vi "UR5 Dash Commands Test VI.vi"() -> ()   [LabVIEW 2018]
panel:
  in  "Command":string="Load target1.urp"
  in  "Send Command":bool
  in  "Get Loaded Program":bool
  in  "Program Name":string="Load target1.urp"
  in  "Stop Program":bool
  in  "Pause":bool
  in  "Play":bool
  in  "Load Program":bool
  in  "Stop":bool
  out "after substring":string
  out "data out":string
  out "Error Out":errorcluster
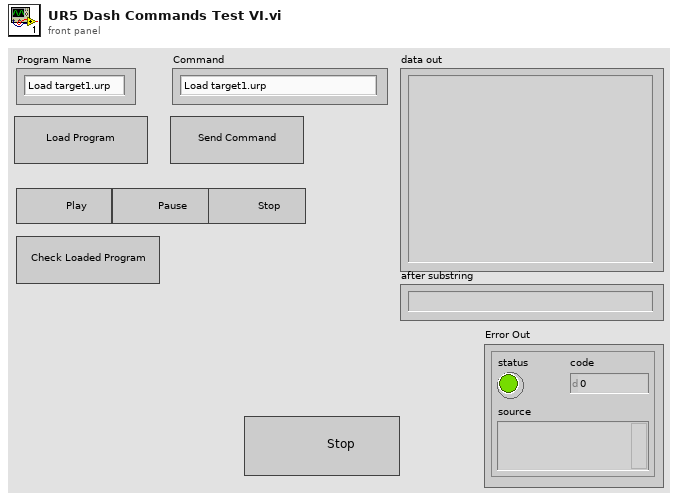
[diagram p1: front panel]
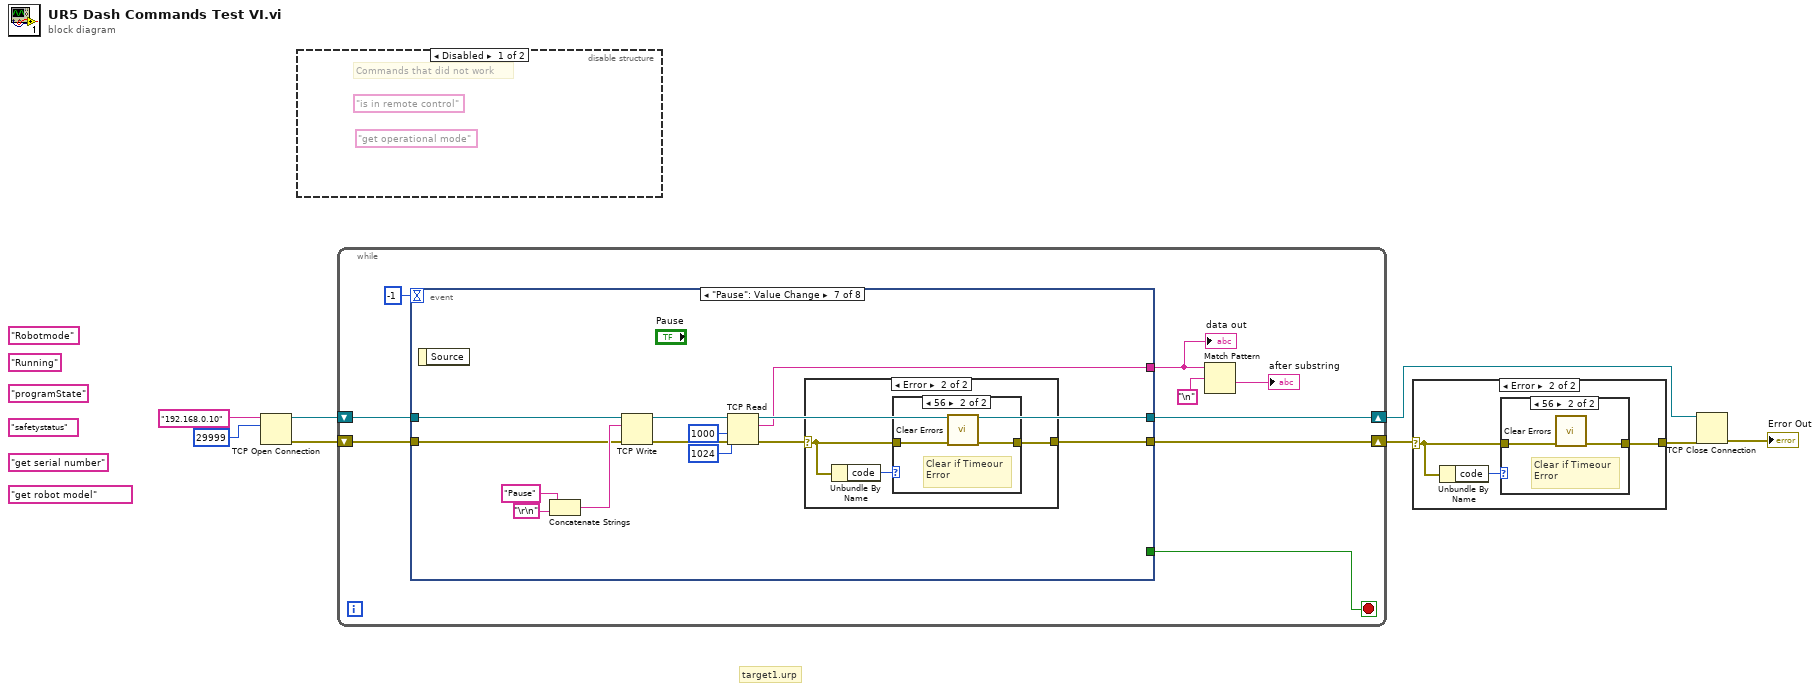
[diagram p0: block diagram]
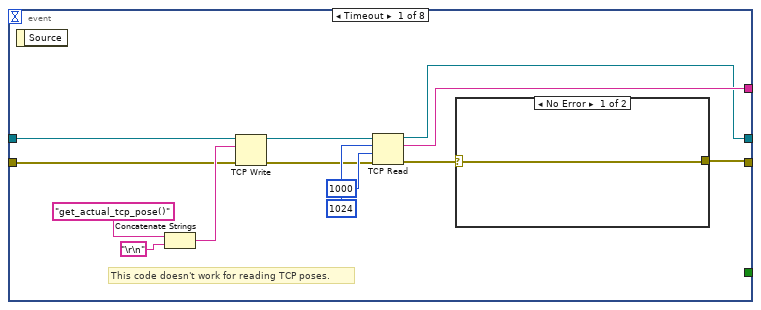
[diagram p4: hidden frame]
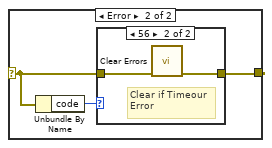
[diagram p5: hidden frame]
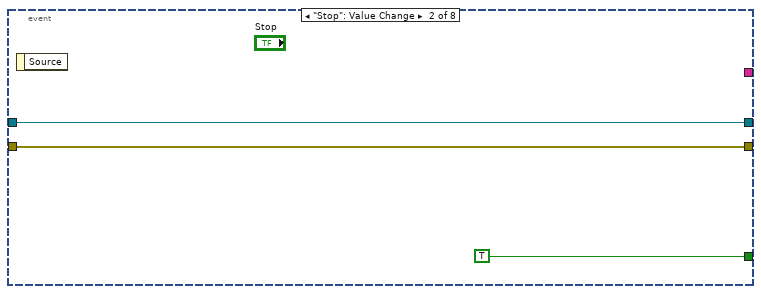
[diagram p7: hidden frame]
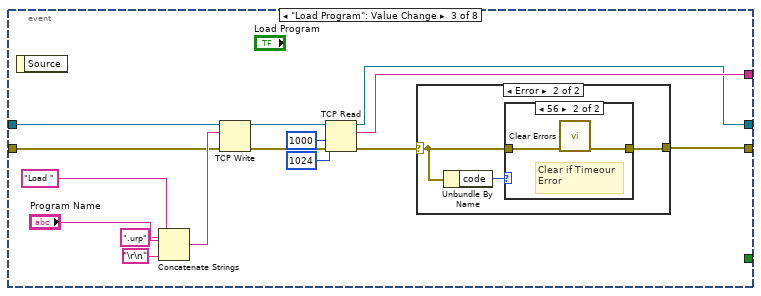
[diagram p8: hidden frame]
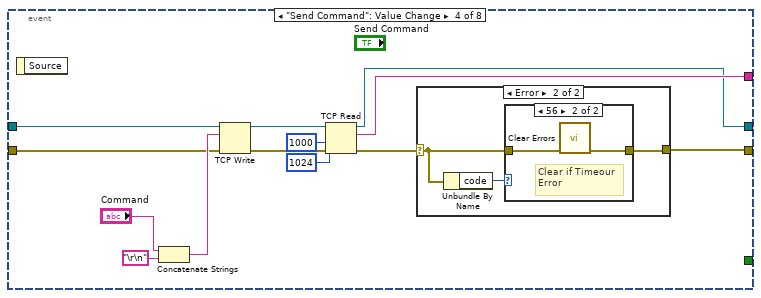
[diagram p11: hidden frame]
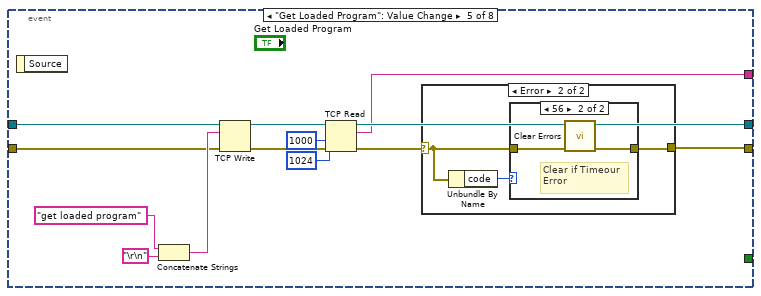
[diagram p14: hidden frame]
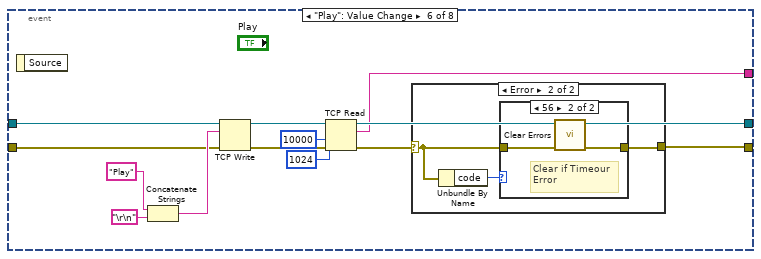
[diagram p17: hidden frame]
diagram:
  (unwired) "Robotmode"
  (unwired) "Running"
  (unwired) "programState"
  (unwired) "safetystatus"
  (unwired) "get serial number"
  (unwired) "get robot model"
  # "target1.urp"
  n1 = TCP Open Connection(address="192.168.0.10", remote port or service name=u16 29999) -> (connection ID=w5:refnum<k5>, error out=w4:errorcluster)  [unwired: 3 in]
  n2 = disable-structure shown="Disabled" {
    frame Disabled {
      (unwired) "get operational mode"
      (unwired) "is in remote control"
      # "Commands that did not work"
    }
    frame Enabled {
    }
  }
  n3 = while {
    shift-right: [w15] -> w1
    shift-left: w5 -> [w16]
    shift-right: [w13] -> w3
    shift-left: w4 -> [w14]
    stop <- w17 stop-if-true
    n4 = event shown="[6] \"Pause\": Value Change" {
      selector: _ -> [_ _ _ _ _ _ _ _]
      dyn-events: _ -> [_ _ _ _ _ _ _ _]
      timeout: -1 -> [_ _ _ _ _ _ _ _]
      tunnel: [_ TRUE _ _ _ _ _ _] -> w17
      tunnel: w16 -> [w23 w39 w49 w69 w89 w109 w129 w149]
      tunnel: [w18 w39 w41 w64 w88 w108 w128 w148] -> w15
      tunnel: [w20 w38 w42 w65 w83 w104 w123 w144] -> w13
      tunnel: w14 -> [w22 w38 w48 w68 w87 w107 w127 w147]
      tunnel: [w19 _ w47 w67 w86 w106 w125 w146] -> w10
      event Timeout {
        # "This code doesn't work for reading TCP poses."
        n5 = event-data() -> ()  [unwired: 1 in, 1 out]
        n6 = Concatenate Strings("get_actual_tcp_pose()" ("string"), "\r\n") -> (w28:string)
        n7 = TCP Write(connection ID=w23, data in=w28, error in (no error)=w22) -> (connection ID out=w30:refnum<k5>, error out=w21:errorcluster)  [unwired: 1 in, 1 out]
        n8 = TCP Read(connection ID=w30, bytes to read=1024, error in (no error)=w21, 9:1000 ("timeout ms (25000)")) -> (connection ID out=w18:refnum<k5>, data out=w19:string, error out=w29:errorcluster)  [unwired: 1 in]
        n9 = case shown="No Error" w29 {
          selector: w29 -> [w31 w33]
          tunnel: [w31 w32] -> w20
          frame No Error {
          }
          frame Error {
            n10 = Unbundle By Name(w33) -> ("code"=w34:i32)
            n11 = case shown="56" w34 {
              tunnel: w33 -> [w35 w37]
              tunnel: [w35 w36] -> w32
              frame 0, Default {
              }
              frame 56 {
                # "Clear if Timeour\nError"
                n12 = call <vilib>:"Clear Errors.vi"("error in (no error)"=w37) -> ("error out"=w36:errorcluster)  [unwired: 5 in, 1 out]
              }
            }
          }
        }
      }
      event "Stop": Value Change {
        n13 = event-data() -> ()  [unwired: 1 in, 1 out]
      }
      event "Load Program": Value Change {
        n14 = event-data() -> ()  [unwired: 1 in, 1 out]
        n15 = Concatenate Strings("Load ", "Program Name", ".urp" ("string"), "\r\n") -> (w53:string)
        n16 = TCP Write(connection ID=w49, data in=w53, error in (no error)=w48) -> (connection ID out=w51:refnum<k5>, error out=w52:errorcluster)  [unwired: 1 in, 1 out]
        n17 = TCP Read(connection ID=w51, bytes to read=1024, error in (no error)=w52, 9:1000 ("timeout ms (25000)")) -> (connection ID out=w41:refnum<k5>, data out=w47:string, error out=w43:errorcluster)  [unwired: 1 in]
        n18 = case shown="Error" w43 {
          selector: w43 -> [w56 w58]
          tunnel: [w56 w57] -> w42
          frame No Error {
          }
          frame Error {
            n19 = Unbundle By Name(w58) -> ("code"=w59:i32)
            n20 = case shown="56" w59 {
              tunnel: w58 -> [w60 w62]
              tunnel: [w60 w61] -> w57
              frame 0, Default {
              }
              frame 56 {
                # "Clear if Timeour\nError"
                n21 = call <vilib>:"Clear Errors.vi"("error in (no error)"=w62) -> ("error out"=w61:errorcluster)  [unwired: 5 in, 1 out]
              }
            }
          }
        }
      }
      event "Send Command": Value Change {
        n22 = event-data() -> ()  [unwired: 1 in, 1 out]
        n23 = Concatenate Strings("Command", "\r\n") -> (w73:string)
        n24 = TCP Write(connection ID=w69, data in=w73, error in (no error)=w68) -> (connection ID out=w71:refnum<k5>, error out=w72:errorcluster)  [unwired: 1 in, 1 out]
        n25 = TCP Read(connection ID=w71, bytes to read=1024, error in (no error)=w72, 9:1000 ("timeout ms (25000)")) -> (connection ID out=w64:refnum<k5>, data out=w67:string, error out=w66:errorcluster)  [unwired: 1 in]
        n26 = case shown="Error" w66 {
          selector: w66 -> [w76 w78]
          tunnel: [w76 w77] -> w65
          frame No Error {
          }
          frame Error {
            n27 = Unbundle By Name(w78) -> ("code"=w79:i32)
            n28 = case shown="56" w79 {
              tunnel: w78 -> [w80 w82]
              tunnel: [w80 w81] -> w77
              frame 0, Default {
              }
              frame 56 {
                # "Clear if Timeour\nError"
                n29 = call <vilib>:"Clear Errors.vi"("error in (no error)"=w82) -> ("error out"=w81:errorcluster)  [unwired: 5 in, 1 out]
              }
            }
          }
        }
      }
      event "Get Loaded Program": Value Change {
        n30 = event-data() -> ()  [unwired: 1 in, 1 out]
        n31 = Concatenate Strings("get loaded program", "\r\n") -> (w93:string)
        n32 = TCP Write(connection ID=w89, data in=w93, error in (no error)=w87) -> (connection ID out=w91:refnum<k5>, error out=w92:errorcluster)  [unwired: 1 in, 1 out]
        n33 = TCP Read(connection ID=w91, bytes to read=1024, error in (no error)=w92, 9:1000 ("timeout ms (25000)")) -> (connection ID out=w88:refnum<k5>, data out=w86:string, error out=w84:errorcluster)  [unwired: 1 in]
        n34 = case shown="Error" w84 {
          selector: w84 -> [w96 w98]
          tunnel: [w96 w97] -> w83
          frame No Error {
          }
          frame Error {
            n35 = Unbundle By Name(w98) -> ("code"=w99:i32)
            n36 = case shown="56" w99 {
              tunnel: w98 -> [w100 w102]
              tunnel: [w100 w101] -> w97
              frame 0, Default {
              }
              frame 56 {
                # "Clear if Timeour\nError"
                n37 = call <vilib>:"Clear Errors.vi"("error in (no error)"=w102) -> ("error out"=w101:errorcluster)  [unwired: 5 in, 1 out]
              }
            }
          }
        }
      }
      event "Play": Value Change {
        n38 = event-data() -> ()  [unwired: 1 in, 1 out]
        n39 = Concatenate Strings("Play", "\r\n") -> (w113:string)
        n40 = TCP Write(connection ID=w109, data in=w113, error in (no error)=w107) -> (connection ID out=w111:refnum<k5>, error out=w112:errorcluster)  [unwired: 1 in, 1 out]
        n41 = TCP Read(connection ID=w111, bytes to read=1024, error in (no error)=w112, 9:10000 ("timeout ms (25000)")) -> (connection ID out=w108:refnum<k5>, data out=w106:string, error out=w105:errorcluster)  [unwired: 1 in]
        n42 = case shown="Error" w105 {
          selector: w105 -> [w116 w118]
          tunnel: [w116 w117] -> w104
          frame No Error {
          }
          frame Error {
            n43 = Unbundle By Name(w118) -> ("code"=w119:i32)
            n44 = case shown="56" w119 {
              tunnel: w118 -> [w120 w122]
              tunnel: [w120 w121] -> w117
              frame 0, Default {
              }
              frame 56 {
                # "Clear if Timeour\nError"
                n45 = call <vilib>:"Clear Errors.vi"("error in (no error)"=w122) -> ("error out"=w121:errorcluster)  [unwired: 5 in, 1 out]
              }
            }
          }
        }
      }
      event "Pause": Value Change {
        n46 = event-data() -> ()  [unwired: 1 in, 1 out]
        n47 = Concatenate Strings("Pause" ("string"), "\r\n") -> (w133:string)
        n48 = TCP Write(connection ID=w129, data in=w133, error in (no error)=w127) -> (connection ID out=w131:refnum<k5>, error out=w132:errorcluster)  [unwired: 1 in, 1 out]
        n49 = TCP Read(connection ID=w131, bytes to read=1024, error in (no error)=w132, 9:1000 ("timeout ms (25000)")) -> (connection ID out=w128:refnum<k5>, data out=w125:string, error out=w124:errorcluster)  [unwired: 1 in]
        n50 = case shown="Error" w124 {
          selector: w124 -> [w136 w138]
          tunnel: [w136 w137] -> w123
          frame No Error {
          }
          frame Error {
            n51 = Unbundle By Name(w138) -> ("code"=w139:i32)
            n52 = case shown="56" w139 {
              tunnel: w138 -> [w140 w142]
              tunnel: [w140 w141] -> w137
              frame 0, Default {
              }
              frame 56 {
                # "Clear if Timeour\nError"
                n53 = call <vilib>:"Clear Errors.vi"("error in (no error)"=w142) -> ("error out"=w141:errorcluster)  [unwired: 5 in, 1 out]
              }
            }
          }
        }
      }
      event "Stop Program": Value Change {
        n54 = event-data() -> ()  [unwired: 1 in, 1 out]
        n55 = Concatenate Strings("Stop", "\r\n") -> (w153:string)
        n56 = TCP Write(connection ID=w149, data in=w153, error in (no error)=w147) -> (connection ID out=w151:refnum<k5>, error out=w152:errorcluster)  [unwired: 1 in, 1 out]
        n57 = TCP Read(connection ID=w151, bytes to read=1024, error in (no error)=w152, 9:1000 ("timeout ms (25000)")) -> (connection ID out=w148:refnum<k5>, data out=w146:string, error out=w143:errorcluster)  [unwired: 1 in]
        n58 = case shown="Error" w143 {
          selector: w143 -> [w156 w158]
          tunnel: [w156 w157] -> w144
          frame No Error {
          }
          frame Error {
            n59 = Unbundle By Name(w158) -> ("code"=w159:i32)
            n60 = case shown="56" w159 {
              tunnel: w158 -> [w160 w162]
              tunnel: [w160 w161] -> w157
              frame 0, Default {
              }
              frame 56 {
                # "Clear if Timeour\nError"
                n61 = call <vilib>:"Clear Errors.vi"("error in (no error)"=w162) -> ("error out"=w161:errorcluster)  [unwired: 5 in, 1 out]
              }
            }
          }
        }
      }
    }
    "data out" <- w10
    n62 = Match Pattern(string=w10, regular expression="\n") -> (after substring=→"after substring":string)  [unwired: 1 in, 3 out]
  }
  n63 = case shown="Error" w3 {
    selector: w3 -> [w163 w165]
    tunnel: [w163 w164] -> w2
    frame No Error {
    }
    frame Error {
      n64 = Unbundle By Name(w165) -> ("code"=w166:i32)
      n65 = case shown="56" w166 {
        tunnel: w165 -> [w167 w169]
        tunnel: [w167 w168] -> w164
        frame 0, Default {
        }
        frame 56 {
          # "Clear if Timeour\nError"
          n66 = call <vilib>:"Clear Errors.vi"("error in (no error)"=w169) -> ("error out"=w168:errorcluster)  [unwired: 5 in, 1 out]
        }
      }
    }
  }
  n67 = TCP Close Connection(connection ID=w1, error in (no error)=w2) -> (error out=→"Error Out":errorcluster)  [unwired: 1 in, 1 out]
